vi "ForceAngleTo_0_360.vi"(8 "error in (no error)":errorcluster, 9 "Use angle class?":bool=TRUE, 10 "Angle in":dbl, 11 "Angle in":refnum<class "Angle.lvclass">) -> (0 "error out":errorcluster, 2 "Forced Angle":dbl)   [LabVIEW 2013, in "Angle.lvclass"]
doc: "Takes in an angle object or a double (specified with the boolean), and outputs the angle as a double, in between 0-360.\n\nEric Schneider, Feb. 2014"
uses:
  Angle.lvclass
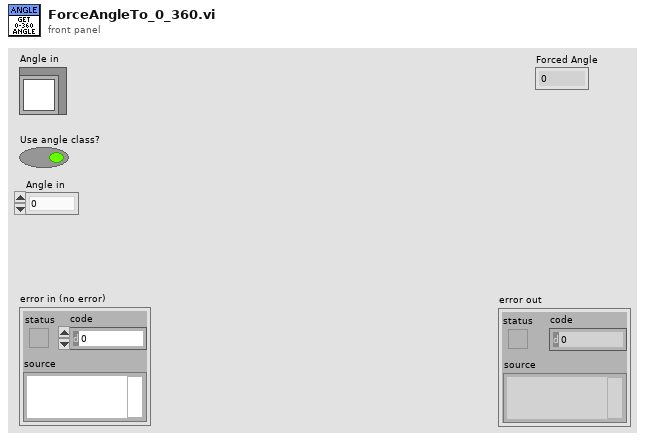
[diagram p1: front panel]
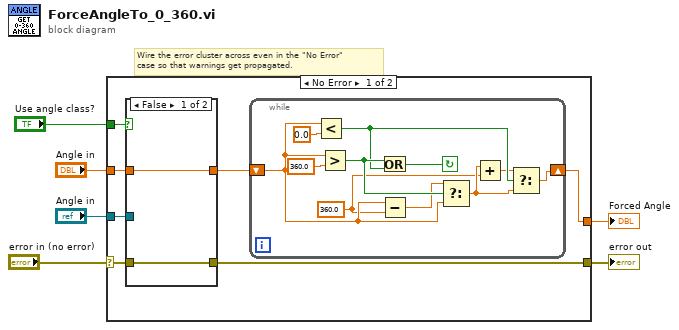
[diagram p0: block diagram]
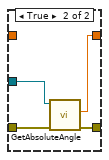
[diagram p2: hidden frame]
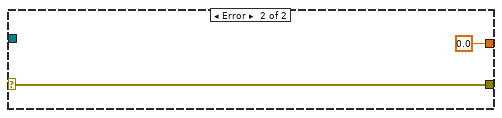
[diagram p3: hidden frame]
diagram:
  # "Wire the error cluster across even in the \"No Error\"\ncase so that warnings get propagated."
  n1 = case shown="No Error" "error in (no error)" {
    selector: "error in (no error)" -> [w12 w32]
    tunnel: [w11 w32] -> w5
    tunnel: "Angle in" -> [w13 _]
    tunnel: [w7 0.0 ("New Angle")] -> w3
    tunnel: "Use angle class?" -> [w10 _]
    tunnel: "Angle in" -> [w9 _]
    frame No Error {
      n2 = case shown="False" w10 {
        tunnel: w13 -> [_ w30]
        tunnel: w12 -> [w25 w29]
        tunnel: [w25 w28] -> w11
        tunnel: [w26 w27] -> w8
        tunnel: w9 -> [w26 _]
        frame False {
        }
        frame True {
          n3 = call "GetAbsoluteAngle.vi"("error in (no error)"=w29, "Angle in"=w30) -> ("error out"=w28:errorcluster, "Absolute angle (Deg.)"=w27:dbl)  [unwired: 8 in]
        }
      }
      n4 = while {
        shift-right: [w14] -> w7
        shift-left: w8 -> [w19]
        stop <- w22 continue-if-true
        w17 = 360.0 ("y")
        n5 = Less?(x=w19, y=0.0) -> (x < y?=w20:bool)
        n6 = Greater?(x=w19, y=360.0) -> (0:w21:bool)
        n7 = Or(x=w21, y=w20) -> (x .or. y?=w22:bool)
        n8 = Subtract(x=w19, y=w17) -> (x-y=w16:dbl)
        n9 = Select(t=w16, s=w21, f=w19) -> (s? t:f=w18:dbl)
        n10 = Add(x=w18, y=w17) -> (x+y=w15:dbl)
        n11 = Select(t=w15, s=w20, f=w18) -> (s? t:f=w14:dbl)
      }
    }
    frame Error {
    }
  }
  "error out" <- w5
  "Forced Angle" <- w3
